vi "4_30_Fxp_addation.vi"(1 "y":fxp<+/-,30,4>, 2 "x":fxp<+/-,30,4>) -> (0 "x+y":fxp<+/-,31,5> format="%.41g")   [LabVIEW 2020]
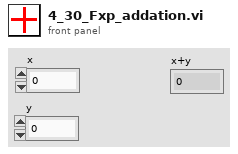
[diagram p1: front panel]
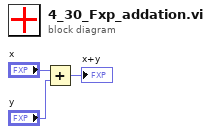
[diagram p0: block diagram]
diagram:
  n1 = Add(x="x", y="y") -> (x+y=→"x+y":fxp<+/-,31,5>)
